vi "Get Resource ID.vi"(4 "UART in":refnum<class "UART.lvclass">) -> (7 "Resource ID":string)   [LabVIEW 2024, in "CTI.lvlib" / "UART.lvclass"]
uses:
  UART.lvclass
  UART.lvclass/UART.ctl
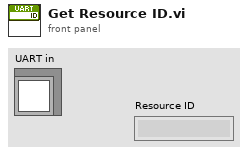
[diagram p1: front panel]
types:
  T1 = typedef "CTI.lvlib/UART Number.ctl" = i8
  T2 = typedef "CTI.lvlib/GPIO Number.ctl" = i8
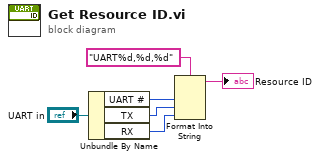
[diagram p0: block diagram]
diagram:
  n1 = Unbundle By Name("UART in") -> ("UART #"=w4:T1, "TX"=w3:T2, "RX"=w2:T2)
  n2 = Format Into String(format string="UART%d,%d,%d", w4, w3, w2) -> (resulting string=→"Resource ID":string)  [unwired: 2 in, 1 out]
